vi "Data_CreateFromFile.vi"(8 "error in (no error)":errorcluster, 11 "Path":path) -> (0 "error out":errorcluster, 2 "data":variant, 3 "success":bool)   [LabVIEW 2017, in "FileManager.lvlib"]
uses:
  <vilib>/addons/InsightCM/Devices/Shared/Common/FileManager/FileManager.lvlib
  <vilib>/addons/InsightCM/Devices/Shared/Common/DataEvent/controls/Event.ctl
  <vilib>/addons/InsightCM/MessageBus/Base/controls/DataEvent.ctl
  <vilib>/addons/InsightCM/MessageBus/Base/controls/KeyValuePair.ctl
  <vilib>/addons/InsightCM/Devices/Shared/Common/DataEvent/controls/DataSet.ctl
  <vilib>/addons/InsightCM/MessageBus/Base/controls/DataSetMetadata.ctl
  <vilib>/addons/InsightCM/MessageBus/Base/controls/TrendPoint.ctl
  <vilib>/addons/InsightCM/MessageBus/Base/controls/TrendAlarmUpdate.ctl
  <vilib>/addons/InsightCM/MessageBus/Base/controls/TrendAlarmTransition.ctl
  <vilib>/addons/InsightCM/Devices/Shared/Common/FileManager/controls/DataPropertyNames.ctl
  <vilib>/addons/InsightCM/Devices/Shared/Common/FileManager/controls/DataType.ctl
  <vilib>/addons/InsightCM/Devices/Shared/Common/DataEvent/DataEvent.lvlib
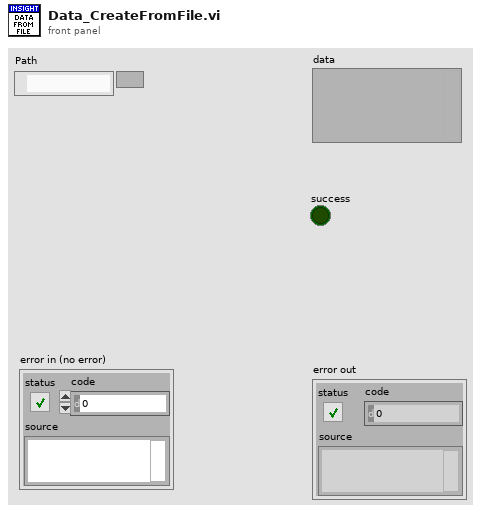
[diagram p1: front panel]
types:
  T1 = typedef "DataEvent.lvlib/Event.ctl" = cluster{"DataEvent":T2, "DataSets":T4[], "TrendPoints":T6[], "Alarms":T7[]}
  T2 = typedef "DataEvent.ctl" = cluster{"Id":string, "AssetNodeId":string, "Timestamp":i64, "Props":T3[]}
  T3 = typedef "KeyValuePair.ctl" = cluster{"Key":string, "Value":string}
  T4 = typedef "DataEvent.lvlib/DataSet.ctl" = cluster{"DataSetMetadata":T5, "Values":sgl[], "Values DVR":refnum<data-value>}
  T5 = typedef "DataSetMetadata.ctl" = cluster{"Id":string, "DataEventId":string, "AssetNodeId":string, "Type":string, "T0":i64, "Props":T3[]}
  T6 = typedef "TrendPoint.ctl" = cluster{"TrendPointId":string, "DataEventId":string, "Timestamp":i64, "Value":dbl, "Props":T3[]}
  T7 = typedef "TrendAlarmUpdate.ctl" = cluster{"RuleId":string, "Transition":T8}
  T8 = typedef "TrendAlarmTransition.ctl" = cluster{"At":i64, "Severity":i32, "Value":dbl}
  T9 = typedef "DataPropertyNames.ctl" = enum16{"Type", "EventRef", "FilePath", "DataGroup", "AcquisitionTimestamp", "StreamId", "StreamBlock", "TrendPointsOnly", "ExtraLargeFile"}
  T10 = typedef "FileManager.lvlib/DataType.ctl" = enum16{"Default", "File", "InMemory", "EventRef", "EventRefFile"}
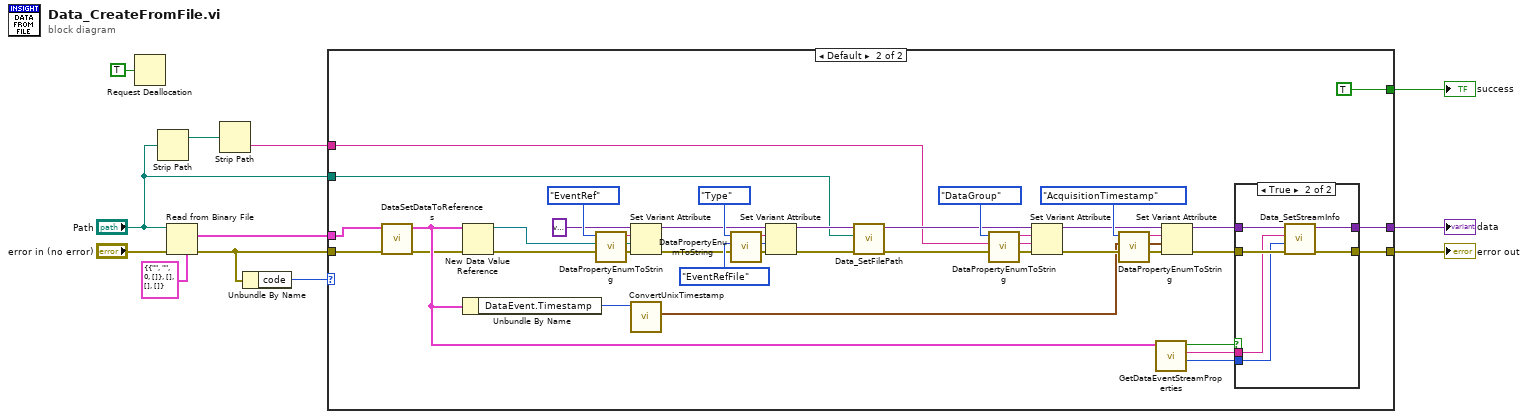
[diagram p0: block diagram]
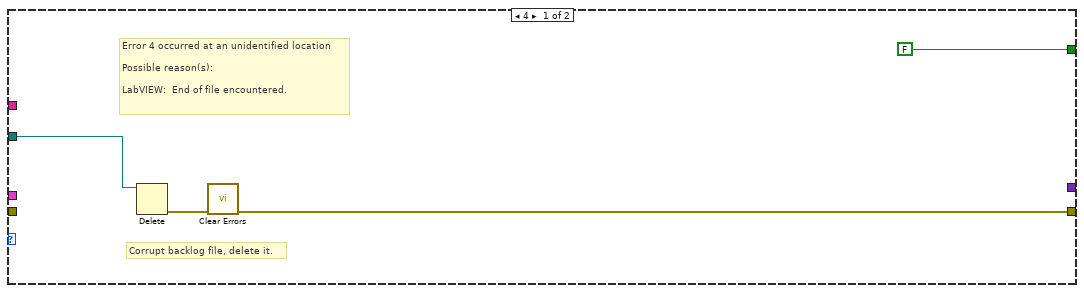
[diagram p2: hidden frame]
diagram:
  n1 = Request Deallocation(TRUE ("flag")) -> ()
  n2 = Strip Path(path="Path") -> (stripped path=w11:path)  [unwired: 1 out]
  n3 = Read from Binary File(5:T1 {"DataEvent"={"Id"="", "AssetNodeId"="", "Timestamp"=0, "Props"=[]}, "DataSets"=[], "TrendPoints"=[], "Alarms"=[]} ("event"), 8:"error in (no error)", 11:"Path") -> (0:w4:errorcluster, 2:w7:T1)  [unwired: 3 in, 2 out]
  n4 = Strip Path(path=w11) -> (name=w9:string)  [unwired: 1 out]
  n5 = Unbundle By Name(w4) -> ("code"=w3:i32)
  n6 = case shown="Default" w3 {
    tunnel: w4 -> [_ w17]
    tunnel: w9 -> [_ w38]
    tunnel: "Path" -> [w15 w29]
    tunnel: w7 -> [_ w19]
    tunnel: [_ w25] -> w6
    tunnel: [w13 w22] -> w5
    tunnel: [FALSE TRUE] -> w2
    frame 4 {
      # "Corrupt backlog file, delete it."
      # "Error 4 occurred at an unidentified location\n\nPossible reason(s):\n\nLabVIEW:  End of file encountered."
      n7 = Delete(path (use dialog)=w15) -> (error out=w14:errorcluster)  [unwired: 4 in, 2 out]
      n8 = call <vilib>:"Clear Errors.vi"("error in (no error)"=w14) -> ("error out"=w13:errorcluster)  [unwired: 5 in, 1 out]
    }
    frame Default {
      n9 = call <vilib>:"DataSetDataToReferences.vi"("error in (no error)"=w17, "data event in"=w19) -> ("error out"=w18:errorcluster, "data event out"=w20:T1)  [unwired: 8 in]
      n10 = New Data Value Reference(data value=w20, error in=w18) -> (data value reference=w33:refnum<data-value>, error out=w44:errorcluster)
      n11 = Unbundle By Name(w20) -> ("DataEvent.Timestamp"=w32:i64)
      n12 = call <vilib>:"DataPropertyEnumToString.vi"("property"=DataPropertyNames."EventRef" ("Names")) -> ("string"=w49:string)  [unwired: 10 in]
      n13 = Set Variant Attribute(Variant=variant ("DataInProgress"), name=w49, value=w33, error in=w44) -> (Variant out=w47:variant, error out=w46:errorcluster)  [unwired: 1 out]
      n14 = call <vilib>:"ConvertUnixTimestamp.vi"("Timestamp in"=w32) -> ("Time Stamp out"=w31:timestamp)  [unwired: 10 in]
      n15 = call <vilib>:"DataPropertyEnumToString.vi"("property"=DataPropertyNames."Type" ("Names")) -> ("string"=w51:string)  [unwired: 10 in]
      n16 = Set Variant Attribute(Variant=w47, name=w51, value=DataType."EventRefFile" ("DataType"), error in=w46) -> (Variant out=w30:variant, error out=w41:errorcluster)  [unwired: 1 out]
      n17 = call <vilib>:"Data_SetFilePath.vi"("error in (no error)"=w41, "path"=w29, "data in"=w30) -> ("error out"=w39:errorcluster, "data out"=w40:variant)  [unwired: 7 in]
      n18 = call <vilib>:"DataPropertyEnumToString.vi"("property"=DataPropertyNames."DataGroup" ("Names")) -> ("string"=w42:string)  [unwired: 10 in]
      n19 = Set Variant Attribute(Variant=w40, name=w42, value=w38, error in=w39) -> (Variant out=w34:variant, error out=w35:errorcluster)  [unwired: 1 out]
      n20 = call <vilib>:"DataPropertyEnumToString.vi"("property"=DataPropertyNames."AcquisitionTimestamp" ("Names")) -> ("string"=w37:string)  [unwired: 10 in]
      n21 = call <vilib>:"GetDataEventStreamProperties.vi"("data event"=w20) -> ("block"=w23:i32, "stream Id"=w24:string, "stream"=w27:bool)  [unwired: 7 in, 1 out]
      n22 = Set Variant Attribute(Variant=w34, name=w37, value=w31, error in=w35) -> (Variant out=w28:variant, error out=w26:errorcluster)  [unwired: 1 out]
      n23 = case shown="True" w27 {
        tunnel: w28 -> [w54 w60]
        tunnel: w26 -> [w53 w59]
        tunnel: [w54 w58] -> w25
        tunnel: [w53 w57] -> w22
        tunnel: w24 -> [_ w56]
        tunnel: w23 -> [_ w55]
        frame False {
        }
        frame True {
          n24 = call <vilib>:"Data_SetStreamInfo.vi"("error in (no error)"=w59, "block"=w55, "streamId"=w56, "data in"=w60) -> ("error out"=w57:errorcluster, "data out"=w58:variant)  [unwired: 6 in]
        }
      }
    }
  }
  "error out" <- w5
  "data" <- w6
  "success" <- w2
